vi "Image_Pixel_Values_GCFS.vi"(5 "Freezing value":sgl, 6 "Temperature":dbl format="%#_13g", 7 "Numeric":i32, 8 "date/time string":string, 10 "Particle messurments":dbl[][](array[numeric]), 11 "Image in":T1) -> (1 "Value_Array":string[](array[string]), 2 "Freezing_points":string[](array[string]), 3 "Freezing data":bool)   [LabVIEW 2024]
uses:
  <vilib>/vision/Image Controls.llb/IMAQ Image.ctl
  <vilib>/vision/NI_Vision_Development_Module.lvlib
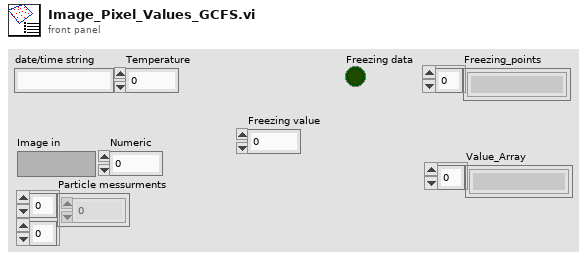
[diagram p1: front panel]
types:
  T1 = typedef "IMAQ Image.ctl" = refnum<image>
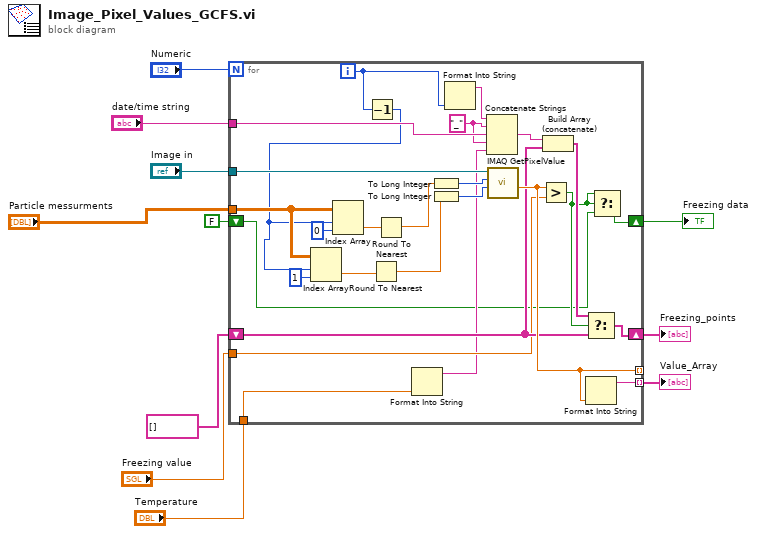
[diagram p0: block diagram]
diagram:
  n1 = for {
    N: "Numeric" -> [_]
    tunnel: "Image in" -> [w38]
    tunnel: [w34] -> _ mode=indexing
    tunnel: [w35] -> w8 mode=indexing
    tunnel: "date/time string" -> [w31]
    shift-right: [w33] -> w9
    shift-left: string[] [] -> [w28]
    tunnel: "Freezing value" -> [w27]
    tunnel: "Temperature" -> [w25]
    tunnel: "Particle messurments" -> [w21]
    shift-right: [w13] -> w2
    shift-left: FALSE -> [w12]
    i -> [w20]
    w26 = "_" ("string")
    n2 = Decrement(x=w20) -> (x-1=w19:i32)
    n3 = Index Array(array=w21, index (row)=w19, index (col)=1) -> (element=w18:dbl)
    n4 = Index Array(array=w21, index (row)=w19, index (col)=0 ("disabled index (col)")) -> (element=w15:dbl)
    n5 = Round To Nearest(number=w18) -> (nearest integer value=w17:dbl)
    n6 = Round To Nearest(number=w15) -> (nearest integer value=w16:dbl)
    n7 = Format Into String(w25) -> (resulting string=w24:string)  [unwired: 3 in, 1 out]
    n8 = To Long Integer(number=w16) -> (32bit integer=w37:i32)
    n9 = To Long Integer(number=w17) -> (32bit integer=w36:i32)
    n10 = Format Into String(w20) -> (resulting string=w32:string)  [unwired: 3 in, 1 out]
    n11 = Concatenate Strings(w32, w26, w31, w26, w24) -> (w30:string)
    n12 = call "IMAQ GetPixelValue"("Image"=w38, "X Coordinate"=w37, "Y Coordinate"=w36) -> ("Pixel Value (Float)"=w34:sgl)  [unwired: 3 in, 4 out]
    n13 = Greater?(x=w34, y=w27) -> (0:w14:bool)
    n14 = Build Array (concatenate)(w30, w28) -> (w29:string[])
    n15 = Select(t=w29, s=w14, f=w28) -> (s? t:f=w33:string[])
    n16 = Format Into String(w34) -> (resulting string=w35:string)  [unwired: 3 in, 1 out]
    n17 = Select(t=w14, s=w14, f=w12) -> (s? t:f=w13:bool)
  }
  "Freezing_points" <- w9
  "Value_Array" <- w8
  "Freezing data" <- w2
